vi "CRYGet Button State.vi"(10 "Channel Name":string, 11 "Input/Output":bool) -> (2 "Exist":bool, 3 "State":T1(ring))   [LabVIEW 2013]
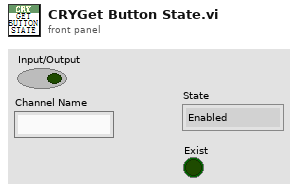
[diagram p1: front panel]
types:
  T1 = enum8{"Enabled", "Disabled", "Disabled and Grayed Out"}
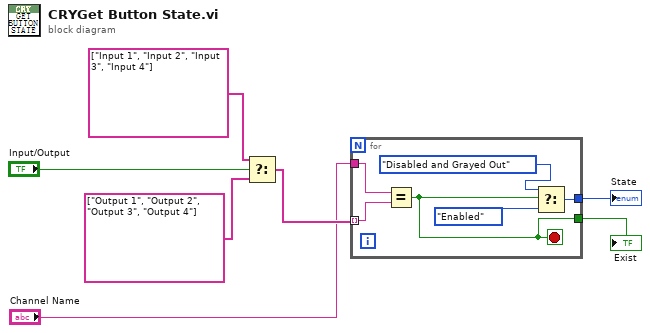
[diagram p0: block diagram]
diagram:
  n1 = Select(t=string[] ["Input 1", "Input 2", "Input 3", "Input 4"], s="Input/Output", f=string[] ["Output 1", "Output 2", "Output 3", "Output 4"]) -> (s? t:f=w4:string[])
  n2 = for {
    tunnel: w4 -> [w12] mode=indexing
    tunnel: "Channel Name" -> [w13]
    tunnel: [w9] -> w2
    tunnel: [w8] -> w1
    stop <- w8 stop-if-true
    n3 = Equal?(x=w13, y=w12) -> (x = y?=w8:bool)
    n4 = Select(t=T1."Disabled and Grayed Out" ("Disabled"), s=w8, f=T1."Enabled") -> (s? t:f=w9:T1)
  }
  "State" <- w2
  "Exist" <- w1
